vi "[RT]SafetyCheck.vi"() -> (3 "No_Error":bool)   [LabVIEW 2018]
uses:
  [GlobVar]SensorState.vi
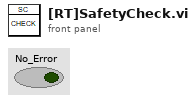
[diagram p1: front panel]
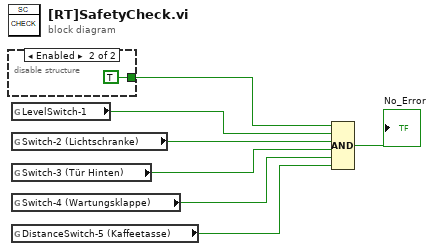
[diagram p0: block diagram]
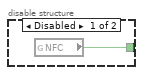
[diagram p2: hidden frame]
diagram:
  n1 = disable-structure shown="Enabled" {
    disable-tunnel: [w8 TRUE ("NFC")] -> w1
    frame Disabled {
      n2 = global read "[GlobVar]SensorState.vi" "NFC"() -> (w8:bool)
    }
    frame Enabled {
    }
  }
  n3 = global read "[GlobVar]SensorState.vi" "LevelSwitch-1"() -> (w2:bool)
  n4 = global read "[GlobVar]SensorState.vi" "Switch-2 (Lichtschranke)"() -> (w3:bool)
  n5 = global read "[GlobVar]SensorState.vi" "Switch-3 (Tür Hinten)"() -> (w4:bool)
  n6 = global read "[GlobVar]SensorState.vi" "Switch-4 (Wartungsklappe)"() -> (w5:bool)
  n7 = global read "[GlobVar]SensorState.vi" "DistanceSwitch-5 (Kaffeetasse)"() -> (w6:bool)
  n8 = Compound Arithmetic op=AND(w1, w2, w3, w4, w5, w6) -> (→"No_Error":bool)
